vi "ConfigSyncInfo.vi"(8 "error in (no error)":errorcluster, 10 "SyncInfo":variant, 11 "NiDaqMx in":refnum<class "NiDaqMx.lvclass">) -> (0 "error out":errorcluster, 3 "NiDaqMx out":refnum<class "NiDaqMx.lvclass">)   [LabVIEW 2014, in "DigitizerPlugins.lvlib" / "NiDaqMx.lvclass"]
uses:
  NiDaqMx.lvclass
  Typedefs/Sync.ctl
  DigitizerBaseClass/DigitizerBase.lvclass/DigitizerBase.ctl
  NiDaqMx.lvclass/NiDaqMx.ctl
  DigitizerBaseClass/Accessors/Write SyncInfo.vi
  DigitizerBaseClass/Accessors/Read SyncInfo.vi
  DigitizerBaseClass/Accessors/Read InstRef.vi
  Accessors/Write OffsetToUtc.vi
  <instrlib>/niSync/niSync.llb/niSync Read Trigger Time Stamp (Single).vi
  <vilib>/DAQmx/read.llb/DAQmx Read (Analog 1D Wfm NChan NSamp).vi
panel:
  out "TrigFracSec":dbl
  out "SampFracSec":dbl
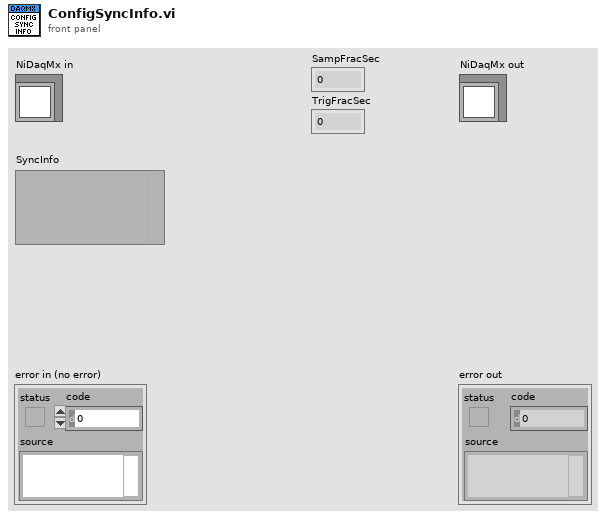
[diagram p1: front panel]
types:
  T1 = typedef "DigitizerPlugins.lvlib/NiDaqMx.lvclass/Sync.ctl" = cluster{"Handle":string, "SrcTerm":string, "DestTerm":string}
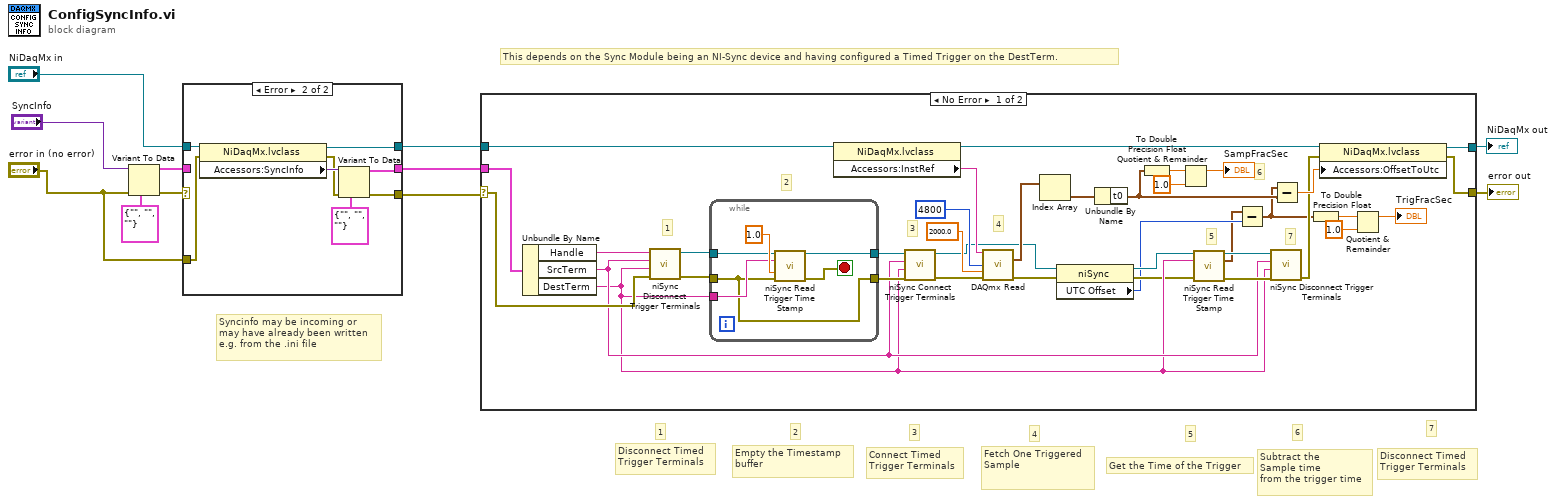
[diagram p0: block diagram]
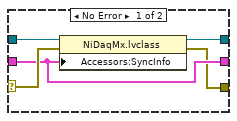
[diagram p2: hidden frame]
diagram:
  # "Syncinfo may be incoming or\nmay have already been written\ne.g. from the .ini file"
  # "Subtract the  \nSample time\nfrom the trigger time"
  # "6"
  # "7"
  # "Disconnect Timed\nTrigger Terminals"
  # "Get the Time of the Trigger"
  # "5"
  # "Fetch One Triggered Sample"
  # "4"
  # "Connect Timed\nTrigger Terminals"
  # "3"
  # "2"
  # "1"
  # "Empty the Timestamp buffer"
  # "Disconnect Timed\nTrigger Terminals"
  # "This depends on the Sync Module being an NI-Sync device and having configured a Timed Trigger on the DestTerm."
  n1 = Variant To Data(error in="error in (no error)", type=T1 {"Handle"="", "SrcTerm"="", "DestTerm"=""} ("Sync"), Variant="SyncInfo") -> (data=w6:T1, error out=w7:errorcluster)
  n2 = case shown="Error" w7 {
    selector: w7 -> [w14 _]
    tunnel: w6 -> [w13 _]
    tunnel: [w16 w20] -> w5
    tunnel: "NiDaqMx in" -> [w15 w21]
    tunnel: [w13 w22] -> w3
    tunnel: [w12 w23] -> w2
    tunnel: "error in (no error)" -> [_ w17]
    frame No Error {
      n3 = property class="NiDaqMx.lvclass"(reference=w15, error in=w14, "Accessors:SyncInfo"=w13) -> (reference out=w16:refnum<class "NiDaqMx.lvclass">, error out=w12:errorcluster)
    }
    frame Error {
      n4 = property class="NiDaqMx.lvclass"(reference=w21, error in=w17) -> (reference out=w20:refnum<class "NiDaqMx.lvclass">, error out=w18:errorcluster, "Accessors:SyncInfo"=w19:variant)
      n5 = Variant To Data(error in=w18, type=T1 {"Handle"="", "SrcTerm"="", "DestTerm"=""} ("Sync"), Variant=w19) -> (data=w22:T1, error out=w23:errorcluster)
    }
  }
  n6 = case shown="No Error" w2 {
    selector: w2 -> [w59 w69]
    tunnel: w5 -> [w54 w68]
    tunnel: w3 -> [w61 _]
    tunnel: [w33 w69] -> w10
    tunnel: [w34 w68] -> w9
    frame No Error {
      # "6"
      # "7"
      # "5"
      # "4"
      # "3"
      # "2"
      # "1"
      n7 = Unbundle By Name(w61) -> ("Handle"=w60:string, "SrcTerm"=w46:string, "DestTerm"=w45:string)
      n8 = call <instrlib>:"niSync Disconnect Trigger Terminals.vi"("error in (no error)"=w59, "destination terminal"=w45, "source terminal"=w46, "instrument handle"=w60) -> ("error out"=w57:errorcluster, "instrument handle out"=w58:refnum<k15>)  [unwired: 6 in]
      n9 = while {
        tunnel: w58 -> [w64]
        tunnel: w57 -> [w62]
        tunnel: [w62] -> w55
        tunnel: [w65] -> w56
        tunnel: w45 -> [w63]
        stop <- w66 stop-if-true
        n10 = call-poly <instrlib>:"niSync Read Trigger Time Stamp.vi"("instrument handle"=w64, "terminal"=w63, "timeout"=1.0, "error in (no error)"=w62) -> ("instrument handle out"=w65:refnum<k15>, "error out"=w66:errorcluster)  [unwired: 8 in, 2 out]
      }
      n11 = property class="NiDaqMx.lvclass"(reference=w54) -> (reference out=w37:refnum<class "NiDaqMx.lvclass">, "Accessors:InstRef"=w53:string)  [unwired: 1 in, 1 out]
      n12 = call <instrlib>:"niSync Connect Trigger Terminals.vi"("error in (no error)"=w55, "destination terminal"=w45, "source terminal"=w46, "instrument handle"=w56) -> ("error out"=w50:errorcluster, "instrument handle out"=w42:refnum<k15>)  [unwired: 6 in]
      n13 = call-poly <vilib>:"DAQmx Read.vi"("task/channels in"=w53, "number of samples per channel"=4800, "timeout"=2000.0, "error in"=w50) -> ("data"=w44:waveform(dbl)[], "error out"=w49:errorcluster)  [unwired: 9 in, 1 out]
      n14 = Index Array(array=w44) -> (element=w39:waveform(dbl))  [unwired: 1 in]
      n15 = property class="niSync"(reference=w42, error in=w49) -> (reference out=w41:refnum<k15>, error out=w43:errorcluster, "UTC Offset"=w40:i32)
      n16 = Unbundle By Name(w39) -> ("t0"=w32:timestamp)
      n17 = To Double Precision Float(number=w32) -> (double precision float=w31:dbl)
      n18 = Quotient & Remainder(x=w31, y=1.0) -> (x-y*floor(x/y)=→"SampFracSec":dbl)  [unwired: 1 out]
      n19 = call-poly <instrlib>:"niSync Read Trigger Time Stamp.vi"("instrument handle"=w41, "terminal"=w45, "error in (no error)"=w43) -> ("instrument handle out"=w47:refnum<k15>, "time stamp out"=w38:timestamp, "error out"=w48:errorcluster)  [unwired: 9 in, 1 out]
      n20 = Subtract(x=w38, y=w40) -> (x-y=w28:timestamp)
      n21 = call <instrlib>:"niSync Disconnect Trigger Terminals.vi"("error in (no error)"=w48, "destination terminal"=w45, "source terminal"=w46, "instrument handle"=w47) -> ("error out"=w35:errorcluster)  [unwired: 6 in, 1 out]
      n22 = Subtract(x=w28, y=w32) -> (x-y=w36:dbl)
      n23 = To Double Precision Float(number=w28) -> (double precision float=w27:dbl)
      n24 = property class="NiDaqMx.lvclass"(reference=w37, error in=w35, "Accessors:OffsetToUtc"=w36) -> (reference out=w34:refnum<class "NiDaqMx.lvclass">, error out=w33:errorcluster)
      n25 = Quotient & Remainder(x=w27, y=1.0) -> (x-y*floor(x/y)=→"TrigFracSec":dbl)  [unwired: 1 out]
    }
    frame Error {
    }
  }
  "error out" <- w10
  "NiDaqMx out" <- w9
